vi "Kelvin Functions be.vi"(2 "n":i32, 3 "x":dbl format="%.2f") -> (1 "ber(x) + bei(x)i":cdb format="%.2f")   [LabVIEW 2010, in "NI_Gmath.lvlib"]
doc: "Computes the complex Kelvin function of the first kind."
uses:
  NI_Gmath.lvlib
  lvanlys.dll
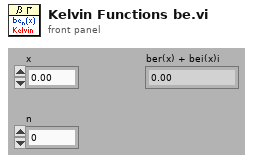
[diagram p1: front panel]
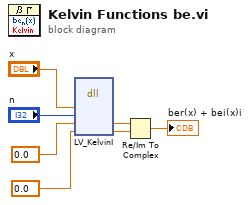
[diagram p0: block diagram]
diagram:
  n1 = dll-call lib="C:/Program Files/National Instruments/LabVIEW 2010/resource/lvanlys.*" fn="LV_KelvinI"("x"="x", "n"="n", "ber"=0.0, "bei"=0.0) -> ("ber"=w3:dbl, "bei"=w2:dbl)  [unwired: 6 in, 2 out]
  n2 = Re/Im To Complex(1:w2, 2:w3) -> (0:→"ber(x) + bei(x)i":cdb)
